vi "Determine if Mouse is in Bounds.vi"(9 "Coords":T1, 11 "XYGraph in":refnum<vi>) -> (3 "In bounds?":bool)   [LabVIEW 2014, in "Graph Extensions.lvlib"]
uses:
  Graph Extensions.lvlib
  <vilib>/Utility/miscctls.llb/LVPoint32TypeDef.ctl
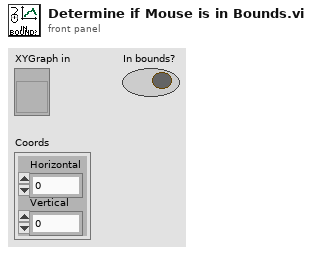
[diagram p1: front panel]
types:
  T1 = typedef "LVPoint32TypeDef.ctl" = cluster{"Horizontal":i32, "Vertical":i32}
  T2 = typedef "LVRectTypeDef.ctl" = cluster{"Left":i16, "Top":i16, "Right":i16, "Bottom":i16}
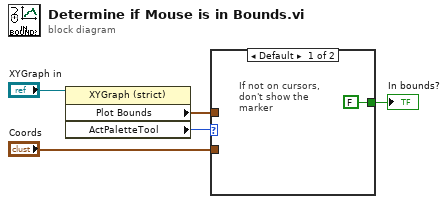
[diagram p0: block diagram]
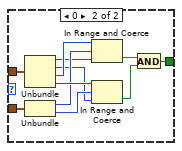
[diagram p2: hidden frame]
diagram:
  n1 = property on="Property Node" class="XYGraph (strict)"(reference="XYGraph in") -> ("Plot Bounds"=w2:T2, "ActPaletteTool"=w1:i32)  [unwired: 1 in, 2 out]
  n2 = case shown="Default" w1 {
    tunnel: [FALSE w17] -> w4
    tunnel: "Coords" -> [_ w16]
    tunnel: w2 -> [_ w7]
    frame Default {
      # "If not on cursors,\ndon't show the \nmarker"
    }
    frame 0 {
      n3 = Unbundle(w7) -> ("Left"=w8:i16, "Top"=w9:i16, "Right"=w12:i16, "Bottom"=w13:i16)
      n4 = Unbundle(w16) -> ("Horizontal"=w11:i32, "Vertical"=w10:i32)
      n5 = In Range and Coerce(upper limit=w12, x=w11, lower limit=w8) -> (In Range?=w14:bool)  [unwired: 1 out]
      n6 = In Range and Coerce(upper limit=w13, x=w10, lower limit=w9) -> (In Range?=w15:bool)  [unwired: 1 out]
      n7 = And(x=w14, y=w15) -> (x .and. y?=w17:bool)
    }
  }
  "In bounds?" <- w4
